vi "Test 1.vi"() -> ()   [LabVIEW 2024]
uses:
  TDMS Data Logger Actor/TDMS Data Logger Actor/TDMS Data Logger Actor.lvclass
  C:/Program Files (x86)/National Instruments/LabVIEW 2024/vi.lib/ActorFramework/Actor/Actor.lvclass
  Data Logger Actor Interface/Data Logger Actor Interface Messages/Start Logging Msg/Start Logging Msg.lvclass/Start Logging Msg.ctl
  <vilib>/ActorFramework/Message Enqueuer/Message Enqueuer.lvclass/Message Enqueuer.ctl
  Data Logger Actor Interface/Data Logger Actor Interface Messages/Log String Data Msg/Log String Data Msg.lvclass/Log String Data Msg.ctl
  Data Logger Actor Interface/Data Logger Actor Interface Messages/Log Double Data Msg/Log Double Data Msg.lvclass/Log Double Data Msg.ctl
  Data Logger Actor Interface/Data Logger Actor Interface Messages/Log Waveform Data Msg/Log Waveform Data Msg.lvclass/Log Waveform Data Msg.ctl
  Data Logger Actor Interface/Data Logger Actor Interface Messages/Set Properties Msg/Set Properties Msg.lvclass/Set Properties Msg.ctl
  <vilib>/ActorFramework/Message Enqueuer/Enqueue.vi
  Data Logger Actor Interface/Data Logger Actor Interface Messages/Start Logging Msg/Start Logging Msg.lvclass
  C:/Program Files (x86)/National Instruments/LabVIEW 2024/vi.lib/ActorFramework/Message/Message.lvclass
  Data Logger Actor Interface/Data Logger Actor Interface Messages/Log String Data Msg/Log String Data Msg.lvclass
  Data Logger Actor Interface/Data Logger Actor Interface Messages/Log Double Data Msg/Log Double Data Msg.lvclass
  Data Logger Actor Interface/Data Logger Actor Interface Messages/Log Waveform Data Msg/Log Waveform Data Msg.lvclass
  Data Logger Actor Interface/Data Logger Actor Interface Messages/Set Properties Msg/Set Properties Msg.lvclass
  Data Logger Actor Interface/Data Logger Actor Interface Messages/Pause Logging Msg/Pause Logging Msg.lvclass
  Data Logger Actor Interface/Data Logger Actor Interface Messages/Resume Logging Msg/Resume Logging Msg.lvclass
  Data Logger Actor Interface/Data Logger Actor Interface Messages/Stop Logging Msg/Stop Logging Msg.lvclass
  <vilib>/ActorFramework/Stop Msg/Stop Msg.lvclass
  <vilib>/ActorFramework/Message Priority Queue/Priority Enqueue.vi
  <vilib>/ActorFramework/Actor/Actor.lvclass
  <vilib>/measure/NI_MABase.lvlib
  C:/Users/uspoaotto/OneDrive - Oregon Tool/Desktop/working copies/dataLogger/TDMS Data Logger Actor/TDMS Data Logger Actor/TDMS Data Logger Actor.lvclass
  C:/Users/uspoaotto/OneDrive - Oregon Tool/Desktop/working copies/dataLogger/Data Logger Actor Interface/Data Logger Actor Interface/Data Logger Actor Interface.lvclass
panel:
  out "Numeric":i32
  # "TEST 1"
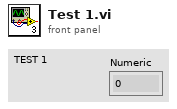
[diagram p1: front panel]
types:
  T1 = enum16{"Sine Wave", "Triangle Wave", "Square Wave", "Sawtooth Wave"}
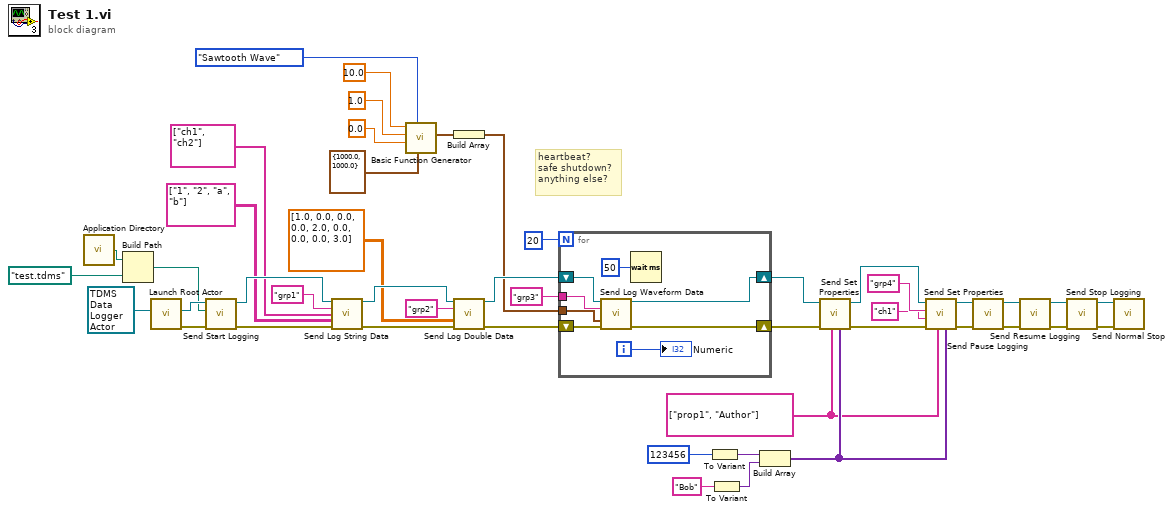
[diagram p0: block diagram]
diagram:
  w17 = string[] ["prop1", "Author"] ("Property Names")
  # "heartbeat?\nsafe shutdown?\nanything else?"
  n1 = call <vilib>:"Application Directory.vi"() -> ("Application Directory"=w40:path)
  n2 = Build Path(base path=w40, name or relative path=path "test.tdms") -> (appended path=w1:path)
  n3 = call <vilib>:"Launch Root Actor.vi"("Actor"=refnum<class "TDMS Data Logger Actor.lvclass"> refnum ("TDMS Data Logger Actor.lvlib:TDMS Data Logger Actor.lvclass")) -> ("error out"=w42:errorcluster, "Actor's Enqueuer"=w45:refnum<class "Message Enqueuer.lvclass">)  [unwired: 9 in]
  n4 = call "Send Start Logging.vi"("error in (no error)"=w42, "Path"=w1, "Message Enqueuer"=w45) -> ("error out"=w5:errorcluster, "Message Enqueuer out"=w44:refnum<class "Message Enqueuer.lvclass">)  [unwired: 7 in]
  n5 = call "Send Log String Data.vi"("Message Enqueuer"=w44, "Group Name (Untitled)"="grp1", "Channel Names (Untitled)"=string[] ["ch1", "ch2"], "Data"=string[][] [["1", "2"], ["a", "b"]], "error in (no error)"=w5) -> ("Message Enqueuer out"=w38:refnum<class "Message Enqueuer.lvclass">, "error out"=w37:errorcluster)  [unwired: 9 in]
  n6 = call <vilib>:"Basic Function Generator.vi"("sampling info"=cluster{"Fs":dbl, "#s":dbl} {"Fs"=1000.0, "#s"=1000.0}, "signal type"=T1."Sawtooth Wave", "phase"=0.0, "amplitude"=1.0, "frequency"=10.0) -> ("signal out"=w34:waveform(dbl))  [unwired: 4 in, 2 out]
  n7 = Build Array(w34) -> (w33:waveform(dbl)[])
  n8 = call "Send Log Double Data.vi"("Message Enqueuer"=w38, "Group Name"="grp2", "Data"=dbl[][] [[1.0, 0.0, 0.0], [0.0, 2.0, 0.0], [0.0, 0.0, 3.0]], "error in (no error)"=w37) -> ("Message Enqueuer out"=w36:refnum<class "Message Enqueuer.lvclass">, "error out"=w35:errorcluster)  [unwired: 10 in]
  n9 = for {
    N: 20 -> [_]
    tunnel: w33 -> [w49]
    tunnel: "grp3" ("Group Name (Untitled)") -> [w48]
    shift-right: [w51] -> w25
    shift-left: w36 -> [w54]
    shift-right: [w52] -> w26
    shift-left: w35 -> [w53]
    i -> [w47]
    n10 = call "Send Log Waveform Data.vi"("Message Enqueuer"=w54, "Group Name (Untitled)"=w48, "Data"=w49, "error in (no error)"=w53) -> ("Message Enqueuer out"=w51:refnum<class "Message Enqueuer.lvclass">, "error out"=w52:errorcluster)  [unwired: 10 in]
    n11 = Wait (ms)(milliseconds to wait=u32 50) -> ()  [unwired: 1 out]
    "Numeric" <- w47
  }
  n12 = To Variant(anything=123456) -> (Variant=w23:variant)
  n13 = To Variant(anything="Bob") -> (Variant=w2:variant)
  n14 = Build Array(w23, w2) -> (w18:variant[])
  n15 = call "Send Set Properties.vi"("Property Values"=w18, "Property Names"=w17, "error in (no error)"=w26, "Message Enqueuer"=w25) -> ("error out"=w21:errorcluster, "Message Enqueuer out"=w22:refnum<class "Message Enqueuer.lvclass">)  [unwired: 6 in]
  n16 = call "Send Set Properties.vi"("Property Values"=w18, "Property Names"=w17, "error in (no error)"=w21, "Channel Name"="ch1", "Group Name"="grp4", "Message Enqueuer"=w22) -> ("error out"=w15:errorcluster, "Message Enqueuer out"=w16:refnum<class "Message Enqueuer.lvclass">)  [unwired: 4 in]
  n17 = call "Send Pause Logging.vi"("error in (no error)"=w15, "Message Enqueuer"=w16) -> ("error out"=w13:errorcluster, "Message Enqueuer out"=w14:refnum<class "Message Enqueuer.lvclass">)  [unwired: 8 in]
  n18 = call "Send Resume Logging.vi"("error in (no error)"=w13, "Message Enqueuer"=w14) -> ("error out"=w12:errorcluster, "Message Enqueuer out"=w11:refnum<class "Message Enqueuer.lvclass">)  [unwired: 8 in]
  n19 = call "Send Stop Logging.vi"("error in (no error)"=w12, "Message Enqueuer"=w11) -> ("error out"=w41:errorcluster, "Message Enqueuer out"=w43:refnum<class "Message Enqueuer.lvclass">)  [unwired: 8 in]
  n20 = call <vilib>:"Send Normal Stop.vi"("error in (no error)"=w41, "Message Enqueuer"=w43) -> ()  [unwired: 9 in, 1 out]
